vi "TimingController.vi"(6 "Duration":u16, 8 "Timer Stop":bool, 9 "Timer Start":bool, 10 "InputGate":bool, 11 "Toggle Modulation On":bool) -> (3 "Running":bool)   [LabVIEW 2019]
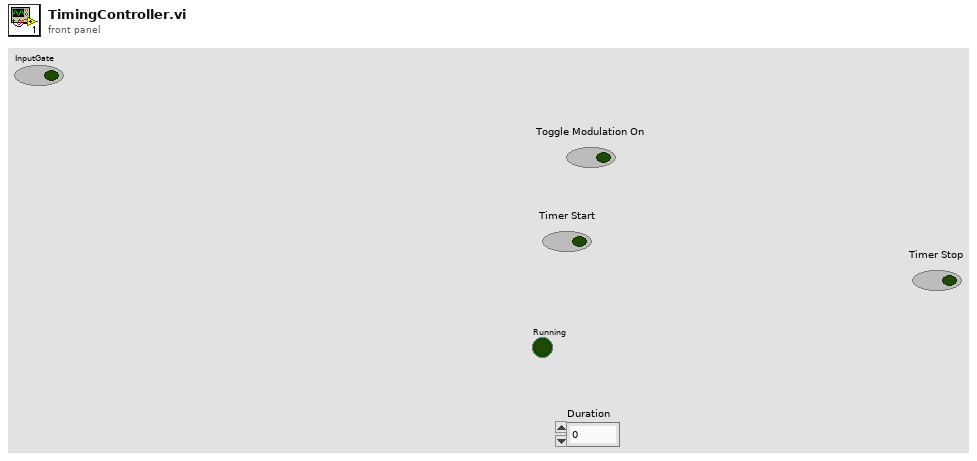
[diagram p1: front panel]
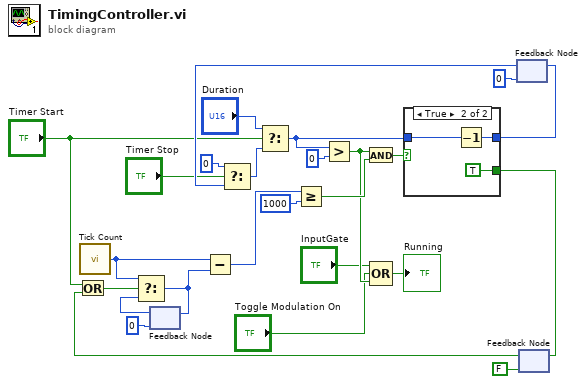
[diagram p0: block diagram]
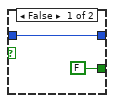
[diagram p2: hidden frame]
diagram:
  n1 = call "Tick Count"() -> ("Tick Count(mSec)"=w22:u32)
  n2 = feedback #1(u32 0 ("Tick Count(mSec)")) -> (w26:u32)
  n3 = feedback #2(u16 0) -> (w9:u16)
  n4 = Select(t=u16 0, s="Timer Stop", f=w9) -> (s? t:f=w8:u16)
  n5 = Select(t="Duration", s="Timer Start", f=w8) -> (s? t:f=w11:u16)
  n6 = Greater?(x=w11, y=u16 0) -> (0:w7:bool)
  n7 = Compound Arithmetic op=OR("InputGate", "Toggle Modulation On", w7) -> (→"Running":bool)
  n8 = feedback #3(FALSE) -> (w18:bool)
  n9 = Or(x="Timer Start", y=w18) -> (x .or. y?=w24:bool)
  n10 = Select(t=w22, s=w24, f=w26) -> (s? t:f=w23:u32)
  n11 = feedback-in #1(w23) -> ()
  n12 = Subtract(x=w22, y=w23) -> (x-y=w21:u32)
  n13 = Greater Or Equal?(x=w21, y=u32 1000) -> (x >= y?=w16:bool)
  n14 = And(x=w7, y=w16) -> (x .and. y?=w14:bool)
  n15 = case shown="True" w14 {
    tunnel: [FALSE TRUE] -> w19
    tunnel: w11 -> [w27 w30]
    tunnel: [w27 w29] -> w13
    frame False {
    }
    frame True {
      n16 = Decrement(x=w30) -> (x-1=w29:u16)
    }
  }
  n17 = feedback-in #2(w13) -> ()
  n18 = feedback-in #3(w19) -> ()
